vi "channel_select.vi"(8 "error in (no error)":errorcluster, 9 "channelType_spectrum":enum16{"SINGLE", "STICHED"}(ring), 10 "channel DUT (index)":i32, 11 "Thorlabs_OSA300_64 in":refnum<class "OSA300.lvclass">) -> (0 "error out":errorcluster, 3 "Thorlabs_OSA300_64 out":refnum<class "OSA300.lvclass">)   [LabVIEW 2010, in "OSA300.lvclass"]
uses:
  OSA300.lvclass
  OSA20X_misc.lvlib
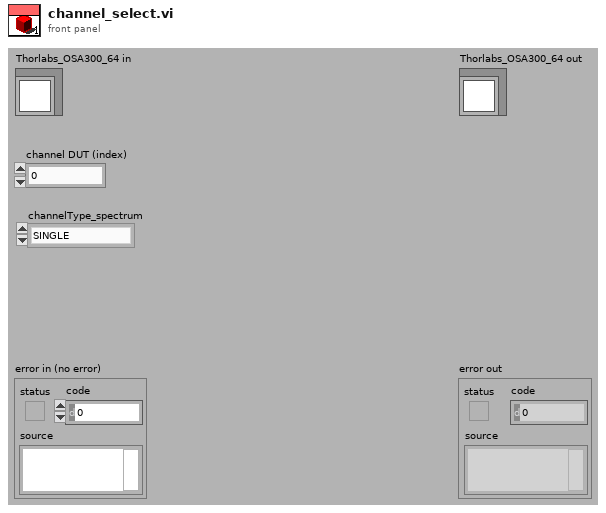
[diagram p1: front panel]
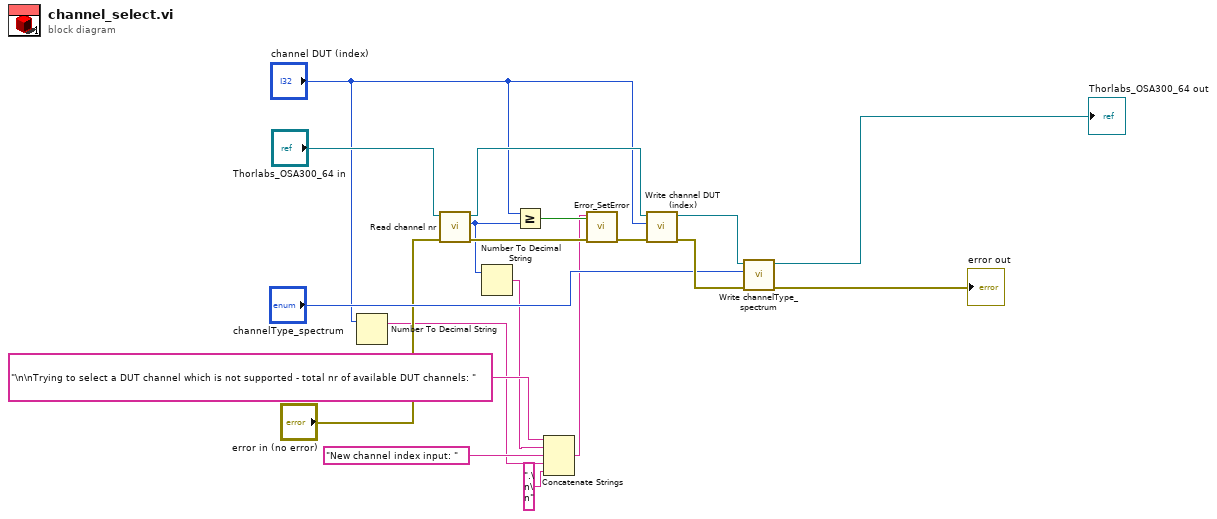
[diagram p0: block diagram]
diagram:
  n1 = Number To Decimal String(number="channel DUT (index)") -> (decimal integer string=w3:string)  [unwired: 1 in]
  n2 = call "Read channel nr.vi"("error in (no error)"="error in (no error)", "OSA300 in"="Thorlabs_OSA300_64 in") -> ("error out"=w11:errorcluster, "channel nr"=w7:i32, "OSA300 out"=w10:refnum<class "OSA300.lvclass">)  [unwired: 7 in]
  n3 = Number To Decimal String(number=w7) -> (decimal integer string=w6:string)  [unwired: 1 in]
  n4 = Greater Or Equal?(x="channel DUT (index)", y=w7) -> (x >= y?=w12:bool)
  n5 = Concatenate Strings("\n\nTrying to select a DUT channel which is not supported - total nr of available DUT channels: " ("source(\"\")"), w6, "New channel index input: " ("string"), w3, ".\n\n" ("string")) -> (w1:string)
  n6 = call "Error_SetError.vi"("error in"=w11, "status (true)"=w12, "source(\"\")"=w1) -> ("error out"=w9:errorcluster)  [unwired: 4 in]
  n7 = call "Write channel DUT (index).vi"("error in (no error)"=w9, "channel DUT (index)"="channel DUT (index)", "OSA300 in"=w10) -> ("error out"=w19:errorcluster, "OSA300 out"=w17:refnum<class "OSA300.lvclass">)  [unwired: 7 in]
  n8 = call "Write channelType_spectrum.vi"("error in (no error)"=w19, "channelType_spectrum"="channelType_spectrum", "OSA300 in"=w17) -> ("error out"=→"error out":errorcluster, "OSA300 out"=→"Thorlabs_OSA300_64 out":refnum<class "OSA300.lvclass">)  [unwired: 7 in]
